vi "Get Conversion Buffers.vi"(8 "error in (no error)":errorcluster, 11 "Transfer Group in":refnum<class "Transfer Group.lvclass">) -> (0 "error out":errorcluster, 1 "string Buffer":refnum<class "Buffer.lvclass">, 2 "engine Buffer":refnum<class "Buffer.lvclass">, 3 "Transfer Group out":refnum<class "Transfer Group.lvclass">)   [LabVIEW 2017, in "DSF Core.lvlib" / "Transfer Group.lvclass"]
uses:
  Transfer Group.lvclass
  Buffer/Buffer.lvclass
  Transfer Group.lvclass/Transfer Group.ctl
  Buffers/Buffers.lvclass
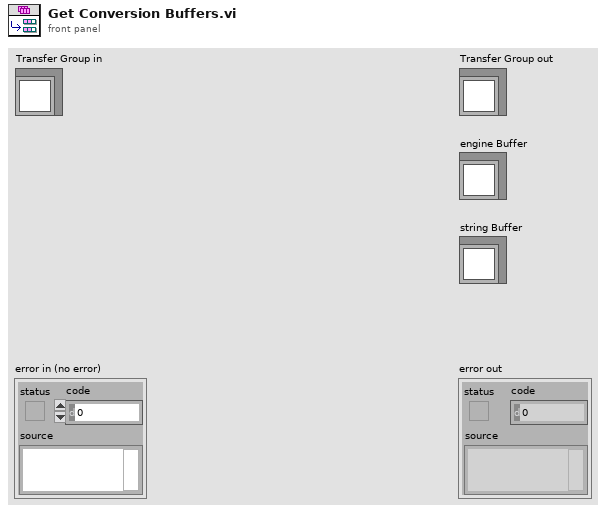
[diagram p1: front panel]
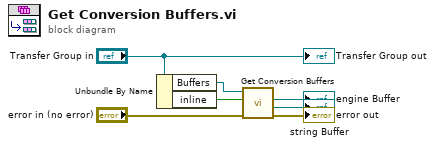
[diagram p0: block diagram]
diagram:
  n1 = Unbundle By Name("Transfer Group in") -> ("Buffers"=w6:refnum<class "Buffers.lvclass">, "inline"=w5:bool)
  n2 = call "Get Conversion Buffers.vi"("error in (no error)"="error in (no error)", "inline?"=w5, "Buffers in"=w6) -> ("error out"=→"error out":errorcluster, "string Buffer"=→"string Buffer":refnum<class "Buffer.lvclass">, "engine Buffer"=→"engine Buffer":refnum<class "Buffer.lvclass">)  [unwired: 5 in, 1 out]
  "Transfer Group out" <- "Transfer Group in"
